vi "Start Profile.vi"(0 "object in":refnum<class "HPS-17000-PowerModule.lvclass">, 11 "Error In":errorcluster) -> (4 "object out":refnum<class "HPS-17000-PowerModule.lvclass">, 15 "Error Out":errorcluster)   [LabVIEW 2023, in "HPS-17000-PowerModule.lvlib" / "HPS-17000-PowerModule.lvclass"]
uses:
  HPS-17000-PowerModule.lvclass
  <instrlib>/HPS-17000/Internal/Start Setpoint Stream Multi.vi
  HPS-17000-PowerModule.lvclass/HPS-17000-PowerModule.ctl
  <instrlib>/HPS-17000/HPS-17000.lvclass
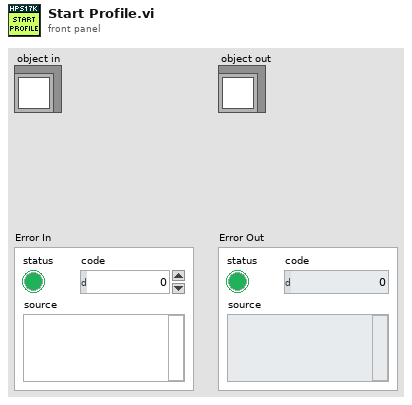
[diagram p1: front panel]
types:
  T1 = typedef "HPS-17000-PowerModule.lvlib/HPS-17000-PowerModule.lvclass/ObjectAttributes.ctl" = cluster{"Configuration":cluster{"TSN NIC IP Address":string, "HPS17000 IP Addresses":string[], "HPS Topology":enum16{"SINGLE", "MULTI"}, "Setpoint Stream Config":T2, "Limits":T3}, "GM ID":string, "HPS17000 Refs":refnum<class "HPS-17000.lvclass">[], "Stream Queues":refnum<queue>[], "connected":bool, "reserved":bool, "events":T4, "nibatterycycler_grpc_Setpoint":T5, "last timestamp":i64, "mode":T6, "range":T7}
  T2 = typedef "Cycler.lvclass/Setpoint Stream Basic Config.ctl" = cluster{"local address":string, "receiver port":u16}
  T3 = typedef "PowerModuleInterface.lvlibp/PowerModuleInterface.lvclass/Limits.ctl" = cluster{"Current Max (A)":dbl, "Current Min (A)":dbl, "Voltage Max (V)":dbl, "Voltage Min (V)":dbl, "Power Max (W)":dbl, "Power Min (W)":dbl}
  T4 = typedef "HPS-17000.lvclass/Multi-Cycler Events.ctl" = cluster{"heartbeats events":refnum<user-event>[], "faults events":refnum<user-event>[], "network sync event":refnum<user-event>[], "setpoint status event":refnum<user-event>[]}
  T5 = typedef "NI_BC_client.lvlib/nibatterycycler_grpc_Setpoint.ctl" = cluster{"voltage":sgl, "current":sgl, "min_power":sgl, "max_power":sgl, "resistance":sgl}
  T6 = typedef "HPS-17000-PowerModule.lvlib/HPS-17000-PowerModule.lvclass/Mode.ctl" = u16
  T7 = typedef "PowerModuleInterface.lvlibp/PowerModuleInterface.lvclass/Range.ctl" = cluster{"Current Max (A)":dbl, "Current Min (A)":dbl, "Voltage Max (V)":dbl, "Voltage Min (V)":dbl}
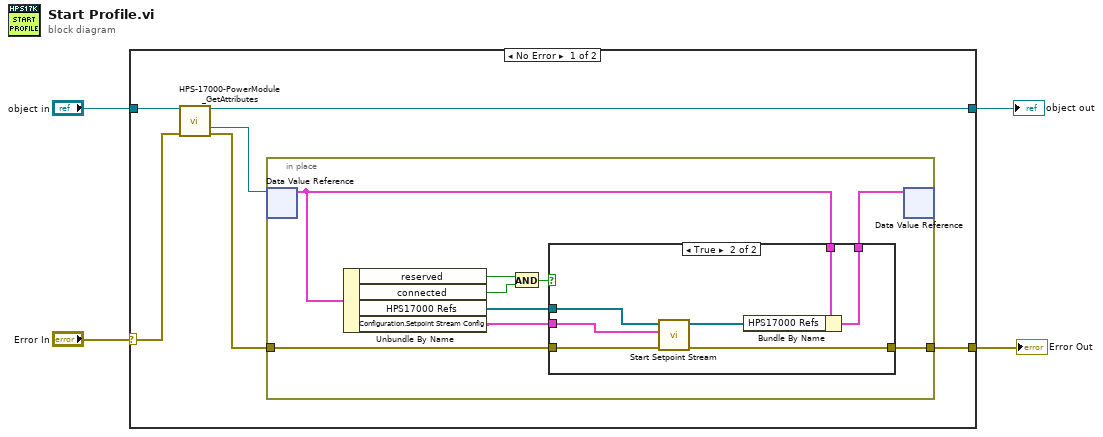
[diagram p0: block diagram]
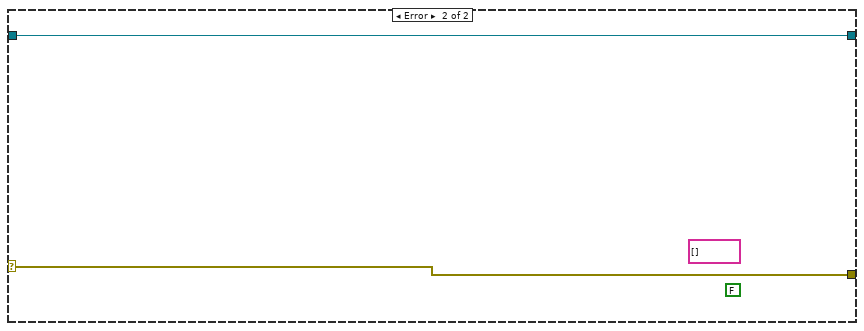
[diagram p3: hidden frame]
diagram:
  n1 = case shown="No Error" "Error In" {
    selector: "Error In" -> [w9 w29]
    tunnel: "object in" -> [w10 w30]
    tunnel: [w5 w30] -> w2
    tunnel: [w6 w29] -> w1
    frame No Error {
      n2 = call "HPS-17000-PowerModule_GetAttributes.vi"("reference in"=w10, "Error In"=w9) -> ("reference out"=w5:refnum<class "HPS-17000-PowerModule.lvclass">, "DataRef"=w8:refnum<data-value>, "Error Out"=w7:errorcluster)  [unwired: 10 in, 1 out]
      n3 = in-place {
        in-place-border: w7 -> [w17]
        in-place-border: [w16] -> w6
        n4 = in-place-dvr #1(w8) -> (w18:T1)  [unwired: 1 out]
        n5 = Unbundle By Name(w18) -> ("reserved"=w13:bool, "connected"=w14:bool, "HPS17000 Refs"=w15:refnum<class "HPS-17000.lvclass">[], "Configuration.Setpoint Stream Config"=w11:T2)
        n6 = And(x=w13, y=w14) -> (x .and. y?=w12:bool)
        n7 = case shown="True" w12 {
          tunnel: [w21 w28] -> w19
          tunnel: w18 -> [w21 w27]
          tunnel: w17 -> [w20 w26]
          tunnel: [w20 w25] -> w16
          tunnel: w15 -> [_ w24]
          tunnel: w11 -> [_ w22]
          frame False {
          }
          frame True {
            n8 = call-poly <instrlib>:"Start Setpoint Stream.vi"("error in"=w26, "setpoint stream config"=w22, "cycler refs in"=w24) -> ("error out"=w25:errorcluster, "cycler refs out"=w23:refnum<class "HPS-17000.lvclass">[])  [unwired: 7 in]
            n9 = Bundle By Name(cluster=w27, "HPS17000 Refs"=w23) -> (w28:T1)
          }
        }
        n10 = in-place-dvr #1(w19) -> ()  [unwired: 2 out]
      }
    }
    frame Error {
      (unwired) string[] []
      (unwired) FALSE
    }
  }
  "Error Out" <- w1
  "object out" <- w2
